vi "hydrolysis_reactor.vi"(2 "#":i16, 4 "Dataflow In":errorcluster) -> (1 "Dataflow Out":errorcluster)   [LabVIEW 2019]
uses:
  lib/libSimulationControl/libSimulationControl.lvlib
panel:
  out "Repetition?":bool
  out "target":path
  out "source":path
  out "prior_active_element":string
  # "*******************************************************************\nBiogas Plant Control\n\nAuthor: Paul Zügel\nGCSC-Frankfurt am Main 2020\n\n*******************************************************************"
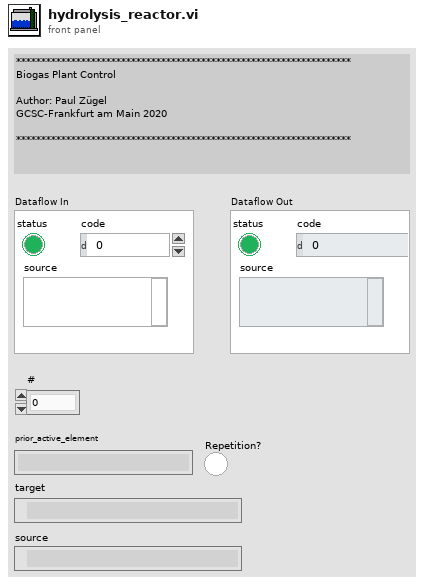
[diagram p1: front panel]
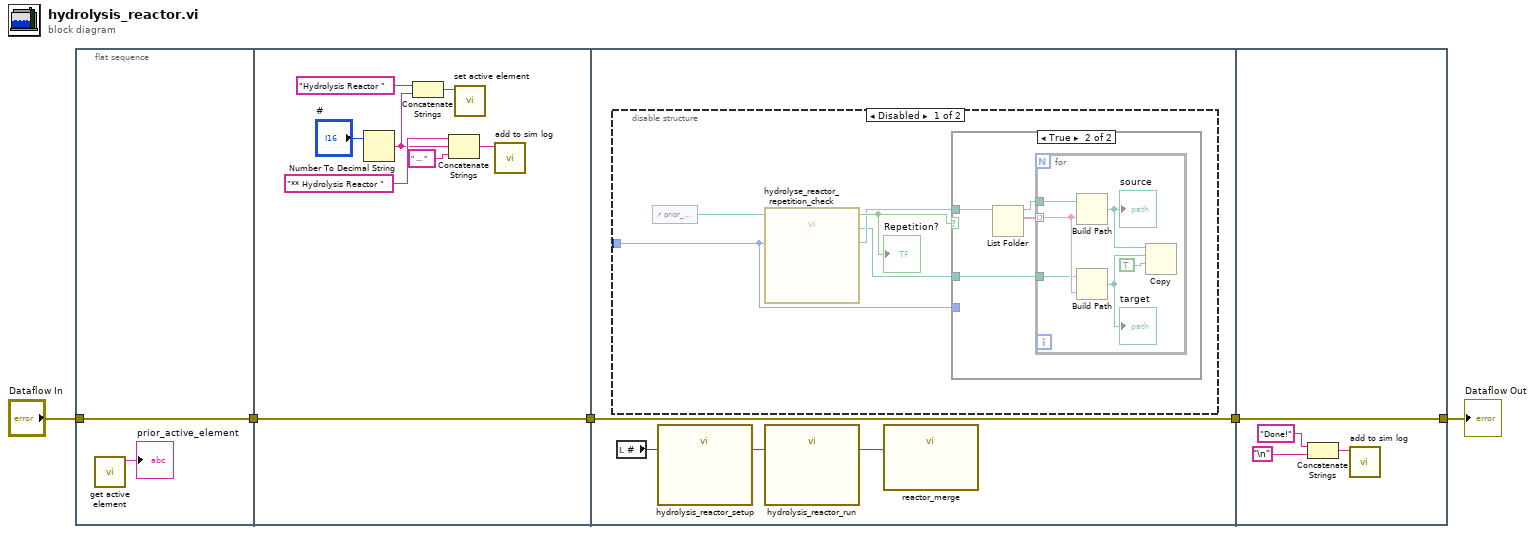
[diagram p0: block diagram]
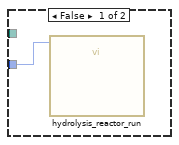
[diagram p2: hidden frame]
diagram:
  n1 = flat-sequence {
    tunnel: "Dataflow In" -> [w7]
    tunnel: [w7] -> w2
    tunnel: [w15] -> w4
    tunnel: w2 -> [w15]
    tunnel: [w19] -> w1
    tunnel: w4 -> [w19]
    tunnel: [w39] -> w3
    tunnel: w1 -> [w39]
    frame #0 {
      n2 = call "get active element.vi"() -> ("active_element"=→"prior_active_element":string)  [unwired: 10 in, 1 out]
    }
    frame #1 {
      n3 = Number To Decimal String(number="#") -> (decimal integer string=w11:string)  [unwired: 1 in]
      n4 = Concatenate Strings("Hydrolysis Reactor " ("elem"), w11) -> (w13:string)
      n5 = Concatenate Strings("** Hydrolysis Reactor " ("string"), w11, " ... " ("string")) -> (w9:string)
      n6 = call "set active element.vi"("elem"=w13) -> ()  [unwired: 10 in, 1 out]
      n7 = call "add to sim log.vi"("log"=w9) -> ()  [unwired: 10 in, 1 out]
    }
    frame #2 {
      n8 = disable-structure shown="Disabled" {
        disable-tunnel: _ -> [w20 _]
        frame Disabled {
          n9 = control-ref of="prior_active_element"() -> (w24:refnum<vi>)
          n10 = call "hydrolyse_reactor_repetition_check.vi"("#"=w20, "Prior Reactor"=w24) -> ("Prior Path"=w22:path, "Current Path"=w21:path, "Repetition?"=w23:bool)  [unwired: 7 in]
          "Repetition?" <- w23
          n11 = case shown="True" w23 {
            tunnel: w20 -> [w25 _]
            tunnel: w22 -> [_ w27]
            tunnel: w21 -> [_ w26]
            frame False {
              n12 = call "hydrolysis_reactor_run.vi"(11:w25) -> ()  [unwired: 10 in, 1 out]
            }
            frame True {
              n13 = List Folder(path=w27) -> (path out=w28:path, filenames=w29:string[])  [unwired: 3 in, 2 out]
              n14 = for {
                tunnel: w29 -> [w34] mode=indexing
                tunnel: w28 -> [w35]
                tunnel: w26 -> [w30]
                n15 = Build Path(base path=w35, name or relative path=w34) -> (appended path=w32:path)
                "source" <- w32
                n16 = Build Path(base path=w30, name or relative path=w34) -> (appended path=w31:path)
                "target" <- w31
                n17 = Copy(9:TRUE ("overwrite (F)"), 10:w31, 11:w32) -> ()  [unwired: 2 in, 3 out]
              }
            }
          }
        }
        frame Enabled {
        }
      }
      n18 = local read "#"() -> (w18:i16)
      n19 = call "hydrolysis_reactor_setup.vi"("#"=w18) -> ("spec_file"=w17:path)  [unwired: 10 in]
      n20 = call "hydrolysis_reactor_run.vi"("spec_file"=w17) -> ("hydrolysis_path"=w16:path)  [unwired: 10 in]
      n21 = call "reactor_merge.vi"("reactor_path"=w16) -> ()  [unwired: 11 in]
    }
    frame #3 {
      n22 = Concatenate Strings("Done!" ("string"), "\n") -> (w36:string)
      n23 = call "add to sim log.vi"("log"=w36) -> ()  [unwired: 10 in, 1 out]
    }
  }
  "Dataflow Out" <- w3
